vi "Get Label.vi"(8 "error in (no error)":errorcluster, 10 "Label":string, 11 "Registry Variant Accessor in":refnum<class "CConfig Variant Accessor.lvclass">) -> (0 "error out":errorcluster, 2 "Valid?":bool, 3 "Registry Variant Accessor out":refnum<class "CConfig Variant Accessor.lvclass">, 5 "Section out":string, 6 "Complete label":string, 7 "Key out":string)   [LabVIEW 2013, in "CConfig Variant Accessor.lvclass"]
doc: "Copyright 2018, Carya Automatisering, Wiebe Walstra."
uses:
  CConfig Variant Accessor.lvclass
  CConfig Variant Accessor.lvclass/CConfig Variant Accessor.ctl
  <vilib>/regexp/Match Regular Expression.xnode
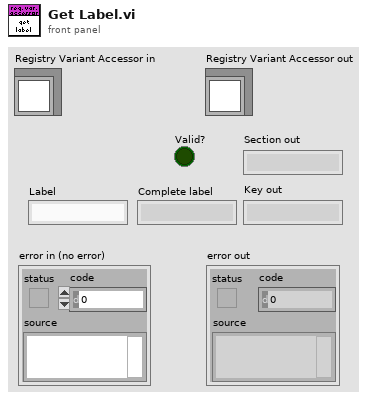
[diagram p1: front panel]
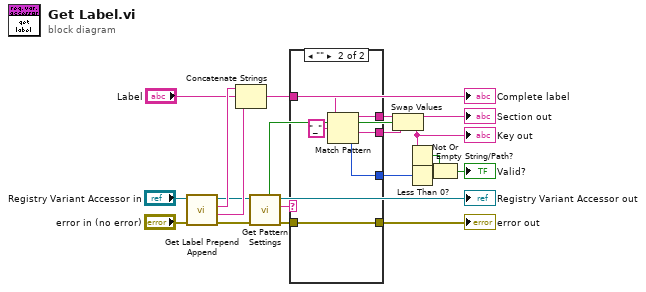
[diagram p0: block diagram]
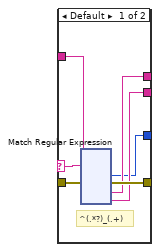
[diagram p2: hidden frame]
diagram:
  n1 = call "Get Label Prepend Append.vi"("error in (no error)"="error in (no error)", "CConfig Variant Accessor in"="Registry Variant Accessor in") -> ("error out"=w10:errorcluster, "Label Append"=w20:string, "Label Prepend"=w21:string, "CConfig Variant Accessor out"=w4:refnum<class "CConfig Variant Accessor.lvclass">)  [unwired: 6 in]
  n2 = Concatenate Strings(w21, "Label", w20) -> (w12:string)
  "Complete label" <- w12
  n3 = call "Get Pattern Settings.vi"("error in (no error)"=w10, "CConfig Variant Accessor in"=w4) -> ("error out"=w5:errorcluster, "Pattern [section_key]"=w1:string, "CConfig Variant Accessor out"=→"Registry Variant Accessor out":refnum<class "CConfig Variant Accessor.lvclass">, "Swap match"=w2:bool)  [unwired: 6 in]
  n4 = case shown="\"\"" w1 {
    selector: w1 -> [w22 _]
    tunnel: [w23 w151] -> w14
    tunnel: [w25 w149] -> w9
    tunnel: [w24 w148] -> w7
    tunnel: w12 -> [w26 w147]
    tunnel: [w28 w146] -> w11
    tunnel: w5 -> [w27 w146]
    frame Default {
      # "^(.*?)_(.+)"
      n5 = xnode "Match Regular Expression"("input string"=w26, "regular expression"=w22, "error in"=w27) -> ("offset past match"=w23:i32, "error out"=w28:errorcluster, "submatch 1"=w25:string, "submatch 2"=w24:string)  [unwired: 3 in, 3 out]
    }
    frame "" {
      n6 = Match Pattern(string=w147, regular expression="_") -> (before substring=w149:string, after substring=w148:string, offset past match=w151:i32)  [unwired: 1 in, 1 out]
    }
  }
  "error out" <- w11
  n7 = Swap Values(12:w9, 13:w2, 14:w7) -> (1:→"Section out":string, 3:w6:string)
  "Key out" <- w6
  n8 = Empty String/Path?(string/path=w6) -> (empty?=w16:bool)
  n9 = Less Than 0?(x=w14) -> (x < 0?=w15:bool)
  n10 = Not Or(1:w15, 2:w16) -> (0:→"Valid?":bool)
